vi "Location Detection.vi"() -> (2 "Computer Name":string, 3 "Location":T1)   [LabVIEW 2022 SP3]
uses:
  -ScanSystem/Controls/location.ctl
  <vilib>/Utility/xml.llb/Read From XML File(string).vi
  <vilib>/Utility/xml.llb/Write to XML File(string).vi
panel:
  in  "Computer Table":cluster{"Computer Name":string, "Location":T1}[](array[cluster])
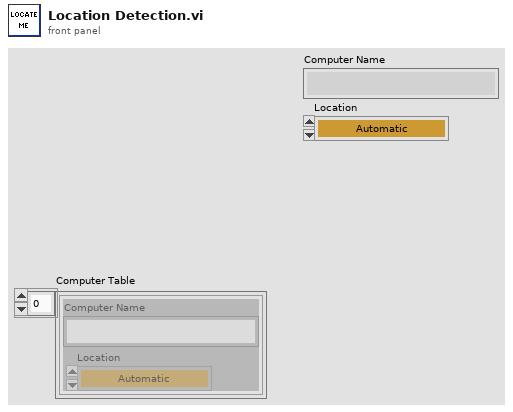
[diagram p1: front panel]
types:
  T1 = typedef "location.ctl" = enum16{"Automatic", "WCM Main", "Hawaii", "Columbia MM3000", "Columbia  NI System", "NYU", "RRI 2", "UHI Allen", "CUMC RT", "Chiba", "Stony Brook", "WCM Microscopy", "WCM Aeoretch", "WCM Optics Lab", "WCM Main 2Axis", "WCM Rotation", "WCM SAM SMAC", "SERI GP"}
  T2 = typedef "ComputerName.ctl" = cluster{"Computer Name":string, "Location":T1}
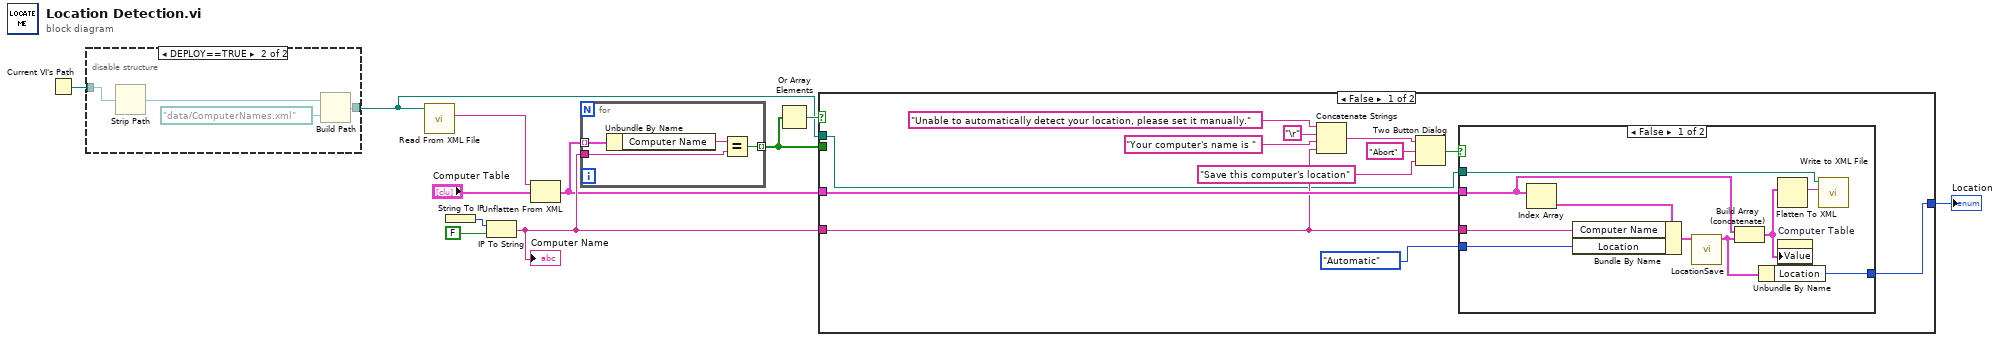
[diagram p0: block diagram]
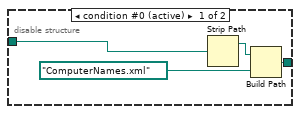
[diagram p2: hidden frame]
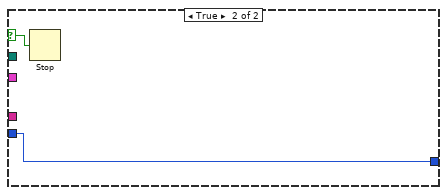
[diagram p3: hidden frame]
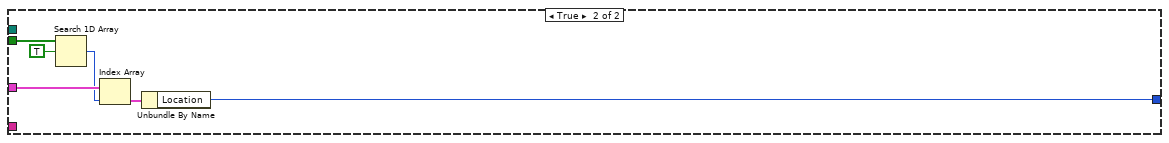
[diagram p4: hidden frame]
diagram:
  n1 = Current VI's Path() -> (path=w2:path)
  n2 = disable-structure shown="DEPLOY==TRUE" {
    disable-tunnel: w2 -> [w15 w17]
    disable-tunnel: [w12 w18] -> w1
    frame condition #0 (active) {
      n3 = Strip Path(path=w15) -> (stripped path=w13:path)  [unwired: 1 out]
      n4 = Build Path(base path=w13, name or relative path=path "ComputerNames.xml" ("path to XML document")) -> (appended path=w12:path)
    }
    frame condition #1 {
      n5 = Strip Path(path=w17) -> (stripped path=w16:path)  [unwired: 1 out]
      n6 = Build Path(base path=w16, name or relative path=path "data/ComputerNames.xml" ("path to XML document")) -> (appended path=w18:path)
    }
  }
  n7 = call-poly <vilib>:"Read From XML File.vi"("XML File Path"=w1) -> ("XML Elements"=w5:string)  [unwired: 8 in, 2 out]
  n8 = String To IP() -> (0:w11:u32)  [unwired: 1 in]
  n9 = IP To String(1:FALSE ("dot notation? (F)"), 2:w11) -> (0:w9:string)
  "Computer Name" <- w9
  n10 = Unflatten From XML(xml string=w5, type="Computer Table") -> (value=w3:cluster{"Computer Name":string, "Location":T1}[])  [unwired: 1 in, 1 out]
  n11 = for {
    tunnel: w3 -> [w23] mode=indexing
    tunnel: w9 -> [w21]
    tunnel: [w20] -> w6 mode=indexing
    n12 = Unbundle By Name(w23) -> ("Computer Name"=w22:string)
    n13 = Equal?(x=w22, y=w21) -> (x = y?=w20:bool)
  }
  n14 = Or Array Elements(Boolean array=w6) -> (logical OR=w7:bool)
  n15 = case shown="False" w7 {
    tunnel: w9 -> [w27 _]
    tunnel: [w24 w48] -> w8
    tunnel: w6 -> [_ w53]
    tunnel: w3 -> [w28 w51]
    tunnel: w1 -> [w26 _]
    frame False {
      n16 = Concatenate Strings("Unable to automatically detect your location, please set it manually." ("message"), "\r", "Your computer's name is " ("string"), w27) -> (w34:string)
      n17 = Two Button Dialog(message=w34, 1:"Save this computer's location" ("F button name (\"Cancel\")"), 2:"Abort" ("T button name (\"OK\")")) -> (T button?=w29:bool)
      n18 = case shown="False" w29 {
        selector: w29 -> [_ w47]
        tunnel: w28 -> [w44 _]
        tunnel: w27 -> [w42 _]
        tunnel: w26 -> [w39 _]
        tunnel: location."Automatic" ("Location") -> [w38 w46]
        tunnel: [w36 w46] -> w24
        frame False {
          n19 = Index Array(array=w44) -> (element=w43:cluster{"Computer Name":string, "Location":T1})  [unwired: 1 in]
          n20 = Bundle By Name(cluster=w43, "Computer Name"=w42, "Location"=w38) -> (w45:cluster{"Computer Name":string, "Location":T1})
          n21 = call "LocationSave.vi"("Computer Name"=w45) -> ("Computer Name Out"=w37:T2)  [unwired: 10 in]
          n22 = Build Array (concatenate)(w44, w37) -> (w41:T2[])
          n23 = Unbundle By Name(w37) -> ("Location"=w36:T1)
          n24 = Flatten To XML(6:w41) -> (2:w40:string)
          n25 = property on="Computer Table" class="Arr (strict)"("Value"=w41) -> ()  [unwired: 2 in, 2 out]
          n26 = call-poly <vilib>:"Write to XML File.vi"("XML Input"=w40, "XML File Path"=w39) -> ()  [unwired: 7 in, 3 out]
        }
        frame True {
          n27 = Stop(stop? (T)=w47) -> ()
        }
      }
    }
    frame True {
      n28 = Search 1D Array(1D array=w53, element=TRUE) -> (index of element=w50:i32)  [unwired: 1 in]
      n29 = Index Array(array=w51, index=w50) -> (element=w49:cluster{"Computer Name":string, "Location":T1})
      n30 = Unbundle By Name(w49) -> ("Location"=w48:T1)
    }
  }
  "Location" <- w8
